vi "Create Evaluations.vi"(8 "error in (no error)":errorcluster, 11 "IEvaluation in":refnum<class "Harmonics_CHP.lvclass">) -> (0 "error out":errorcluster, 2 "Evaluations Out":T1[](array[typedef]) {"Low Limit" format="%#_13g"; "SI Scaling" items=["femto"=-15, "pico"=-12, "nano"=-9, "micro"=-6, "milli"=-3, "percent"=-2, ""=0, "kilo"=3, "mega"=6, "giga"=9, "tera"=12]}, 3 "IEvaluation out":refnum<class "Harmonics_CHP.lvclass">)   [LabVIEW 2016, in "SeqAuto Evaluations.lvlib" / "Harmonics_CHP.lvclass"]
uses:
  Harmonics_CHP.lvclass
  C:/projects/STS/Common/Sequence Automation/Plugins/SeqAuto IEvaluation.lvlibp/SeqAuto IEvaluation.lvclass
  Plugins/TestStand API Tools (TSAT).lvlibp/Evaluation Actions/Includes/Controls/TSAT Evaluation.ctl
  Plugins/TestStand API Tools (TSAT).lvlibp/Evaluation Actions/Includes/Controls/TSAT Eval SI Unit Scaling.ctl
  Plugins/TestStand API Tools (TSAT).lvlibp/Evaluation Actions/Includes/Controls/TSAT Evaluation Type.ctl
  Harmonics_CHP.lvclass/Harmonics_CHP.ctl
  Read Harmonic.vi
  Read SA Pin.vi
  Write Exported Data Location.vi
  Plugins/SeqAuto IEvaluation.lvlibp/Read Measurement Name.vi
  Plugins/TestStand API Tools (TSAT).lvlibp/Evaluation Actions/TSAT Evaluation Actions.lvlib
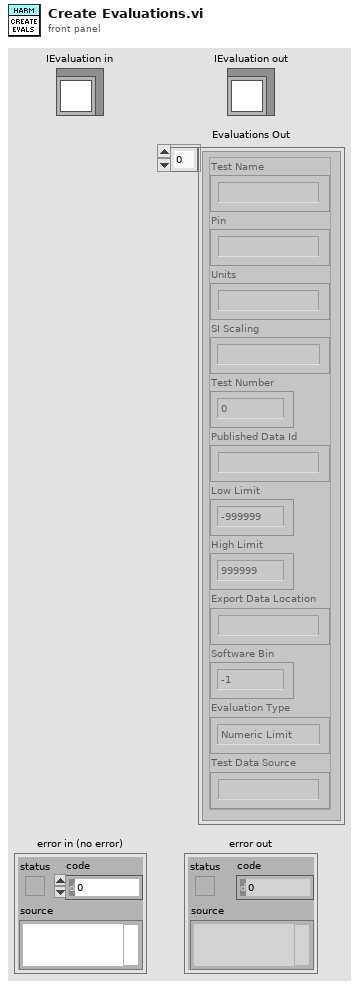
[diagram p1: front panel]
types:
  T1 = typedef "TestStand API Tools (TSAT).lvlibp/TSAT Evaluation Actions.lvlib/TSAT Evaluation.ctl" = cluster{"Test Name":string, "Pin":string, "Units":string, "SI Scaling":T2, "Test Number":i32, "Published Data Id":string, "Low Limit":dbl, "High Limit":dbl, "Export Data Location":string, "Software Bin":i64, "Evaluation Type":T3, "Test Data Source":string}
  T2 = typedef "TestStand API Tools (TSAT).lvlibp/TSAT Evaluation Actions.lvlib/TSAT Eval SI Unit Scaling.ctl" = i16
  T3 = typedef "TestStand API Tools (TSAT).lvlibp/TSAT Evaluation Actions.lvlib/TSAT Evaluation Type.ctl" = enum16{"Numeric Limit", "Pass/Fail", "None"}
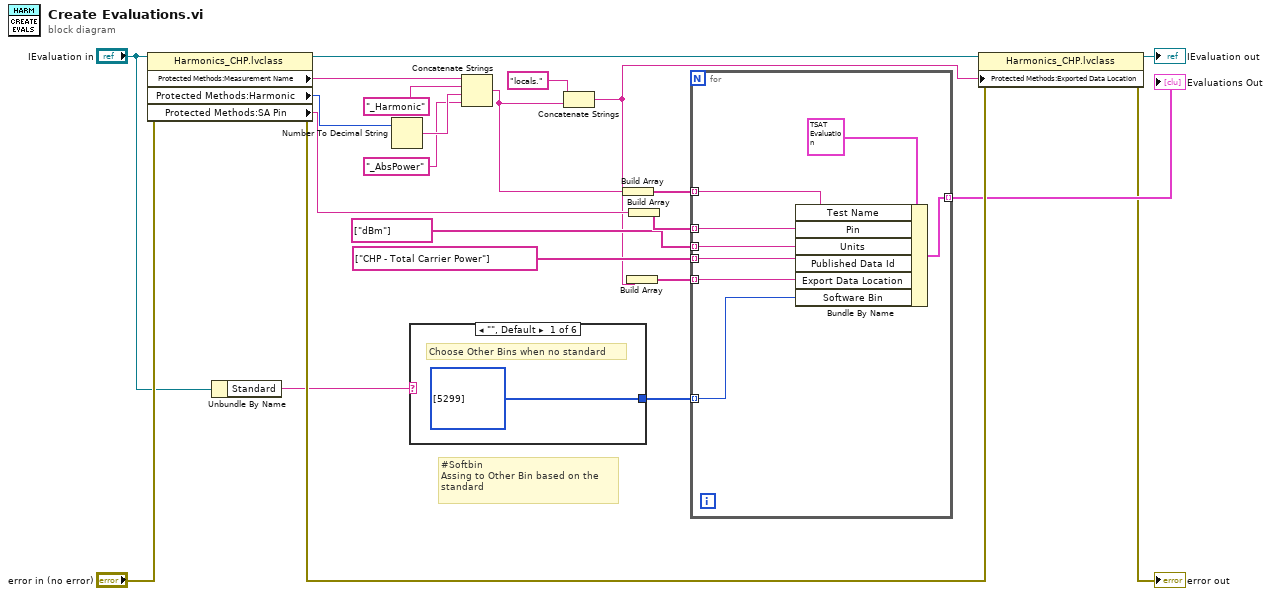
[diagram p0: block diagram]
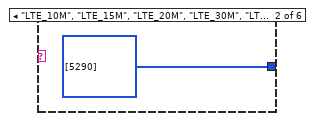
[diagram p2: hidden frame]
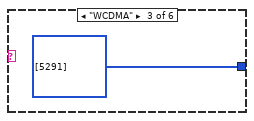
[diagram p3: hidden frame]
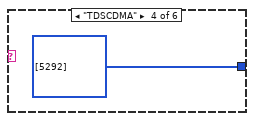
[diagram p4: hidden frame]
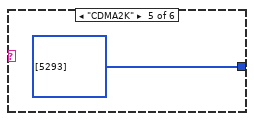
[diagram p5: hidden frame]
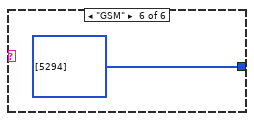
[diagram p6: hidden frame]
diagram:
  # "#Softbin\nAssing to Other Bin based on the \nstandard"
  n1 = property class="Harmonics_CHP.lvclass"(reference="IEvaluation in", error in="error in (no error)") -> (reference out=w9:refnum<class "Harmonics_CHP.lvclass">, error out=w22:errorcluster, "Protected Methods:Measurement Name"=w7:string, "Protected Methods:Harmonic"=w19:i8, "Protected Methods:SA Pin"=w14:string)
  n2 = Unbundle By Name("IEvaluation in") -> ("Standard"=w2:string)
  n3 = Number To Decimal String(number=w19) -> (decimal integer string=w18:string)  [unwired: 1 in]
  n4 = case shown="\"\", Default" w2 {
    tunnel: [i64[] [5299] i64[] [5290] i64[] [5291] i64[] [5292] i64[] [5293] i64[] [5294]] -> w1
    frame "", Default {
      # "Choose Other Bins when no standard"
    }
    frame "LTE_10M", "LTE_15M", "LTE_20M", "LTE_30M", "LTE_40M" {
    }
    frame "WCDMA" {
    }
    frame "TDSCDMA" {
    }
    frame "CDMA2K" {
    }
    frame "GSM" {
    }
  }
  n5 = Concatenate Strings(w7, "_Harmonic" ("string"), w18, "_AbsPower" ("string")) -> (w5:string)
  n6 = Concatenate Strings("locals." ("string"), w5) -> (w4:string)
  n7 = Build Array(w5) -> (w16:string[])
  n8 = Build Array(w4) -> (w15:string[])
  n9 = Build Array(w14) -> (w13:string[])
  n10 = for {
    tunnel: [w36] -> w21 mode=indexing
    tunnel: w16 -> [w35] mode=indexing
    tunnel: w15 -> [w34] mode=indexing
    tunnel: w13 -> [w33] mode=indexing
    tunnel: string[] ["dBm"] -> [w32] mode=indexing
    tunnel: string[] ["CHP - Total Carrier Power"] -> [w31] mode=indexing
    tunnel: w1 -> [w30] mode=indexing
    n11 = Bundle By Name(cluster=T1 {"Test Name"="", "Pin"="", "Units"="", "SI Scaling"=0, "Test Number"=0, "Published Data Id"="", "Low Limit"=-999999.0, "High Limit"=999999.0, "Export Data Location"="", "Software Bin"=-1, "Evaluation Type"=enum."Numeric Limit", "Test Data Source"=""} ("Evaluation"), "Test Name"=w35, "Pin"=w33, "Units"=w32, "Published Data Id"=w31, "Export Data Location"=w34, "Software Bin"=w30) -> (w36:T1)
  }
  "Evaluations Out" <- w21
  n12 = property class="Harmonics_CHP.lvclass"(reference=w9, error in=w22, "Protected Methods:Exported Data Location"=w4) -> (reference out=→"IEvaluation out":refnum<class "Harmonics_CHP.lvclass">, error out=→"error out":errorcluster)
